vi "svx_Polar_Pane_Size.vi"(6 "Container bounds":T1, 7 "Display State In":T2={"Property Name"=[], "Container bounds"={"Width"=550, "Height"=250}, "Scale range"={"Maximum"=1.0, "Increment"=1.0}, "PointIdx"=0, "Marker list"=[], "Color settings"={"Arrow color"=16860, "Magnitude major grid"=13816530, "Magnitude minor grid"=16777216, "Phase grid"=13816530, "Phase scale marker text"=0}, "Magnitude scale name"="Magnitude", "Magnitude scale format string"="%#.2e", "MagnitudeScale:Visible"=TRUE, "MagnitudeScaleLabel:Visible"=TRUE, "PhaseScale:Visible"=TRUE, "Marker:Visible"=TRUE, "Cursor:Visible"=FALSE, "CursorName:Visible"=TRUE, "Autoscale"=TRUE, "Marker color"=16860, "Line color"=16711680, "Cursor color"=16711680, "Magnitude scale marker color"=0, "Plot.Line Style"=0, "Plot.Line Width"=0, "Plot.Point Style"=0, "Cursor.Line Style"=0, "Cursor.Line Width"=0, "Cursor.Point Style"=0, "Cursor.Style"=4, "Marker.Point Style"=2, "Point/fill color"=16711680, "Background color"=16777225, "Cursor name"="", "Cursor Release"=refnum, "Scale Range Change"=refnum, "data size(s)"=[], "Selectors:Visible"=TRUE, "Selector:ring Strings"={"Selector:Custom Strings"=FALSE, "Selector:Row Strings []"=[], "Selector:Column Strings []"=[], "User:Row Strings []"=[], "User:Column Strings []"=[]}, "Lock Cursor Info Position"=FALSE, "CursLoc"={"magnitude"=0.0, "phase"=0.0, "time/rev/RPM"=0.0}, "Plot Area:Position"={"Left"=0, "Top"=0}, "Plot Area:Size"={"Width"=0, "Height"=0}, "Marker.Style"=0, "Indication Arcs"=[], "Arc.Selector"=0, "customized marker"=[], "tree Width"=0, " Parents Tags"=[], "Children Tags"=[], "open?"=[], "index"=[{"row index"=0, "column index"=0}], "Label"="", "custom strings changed"=FALSE, "Owning VI"=refnum, "Legend BG color"=16777225, "Legend font color"=0, "column Width"=203, "attribute"=variant}, 8 "z scale graph Refnum":refnum<vi>, 9 "Plot Legend Refnum":refnum<vi>, 10 "Polar Plot Refnum in":refnum<vi>) -> (0 "z scale graph Refnum out":refnum<vi>, 1 "Plot Legend Refnum out":refnum<vi>, 2 "Polar Plot Refnum out":refnum<vi>, 5 "Display State out":T2={"Property Name"=[], "Container bounds"={"Width"=550, "Height"=250}, "Scale range"={"Maximum"=1.0, "Increment"=1.0}, "PointIdx"=0, "Marker list"=[], "Color settings"={"Arrow color"=16860, "Magnitude major grid"=13816530, "Magnitude minor grid"=16777216, "Phase grid"=13816530, "Phase scale marker text"=0}, "Magnitude scale name"="Magnitude", "Magnitude scale format string"="%#.2e", "MagnitudeScale:Visible"=TRUE, "MagnitudeScaleLabel:Visible"=TRUE, "PhaseScale:Visible"=TRUE, "Marker:Visible"=TRUE, "Cursor:Visible"=FALSE, "CursorName:Visible"=TRUE, "Autoscale"=TRUE, "Marker color"=16860, "Line color"=16711680, "Cursor color"=16711680, "Magnitude scale marker color"=0, "Plot.Line Style"=0, "Plot.Line Width"=0, "Plot.Point Style"=0, "Cursor.Line Style"=0, "Cursor.Line Width"=0, "Cursor.Point Style"=0, "Cursor.Style"=4, "Marker.Point Style"=2, "Point/fill color"=16711680, "Background color"=16777225, "Cursor name"="", "Cursor Release"=refnum, "Scale Range Change"=refnum, "data size(s)"=[], "Selectors:Visible"=TRUE, "Selector:ring Strings"={"Selector:Custom Strings"=FALSE, "Selector:Row Strings []"=[], "Selector:Column Strings []"=[], "User:Row Strings []"=[], "User:Column Strings []"=[]}, "Lock Cursor Info Position"=FALSE, "CursLoc"={"magnitude"=0.0, "phase"=0.0, "time/rev/RPM"=0.0}, "Plot Area:Position"={"Left"=0, "Top"=0}, "Plot Area:Size"={"Width"=0, "Height"=0}, "Marker.Style"=0, "Indication Arcs"=[], "Arc.Selector"=0, "customized marker"=[], "tree Width"=0, " Parents Tags"=[], "Children Tags"=[], "open?"=[], "index"=[{"row index"=0, "column index"=0}], "Label"="", "custom strings changed"=FALSE, "Owning VI"=refnum, "Legend BG color"=16777225, "Legend font color"=0, "column Width"=203, "attribute"=variant} caption="State")   [LabVIEW 2017, in "SVX Polar Plot.xctl"]
uses:
  <vilib>/addons/_XControls/Polar Plot/SVX Polar Plot.xctl
  <vilib>/addons/_XControls/Polar Plot/subVIs/svx_Polar_Plot_Internal_State.ctl
  <vilib>/addons/_XControls/Polar Plot/subVIs/svx_Polar_Indication_Arcs.ctl
  <vilib>/addons/_XControls/Polar Plot/subVIs/svx_Polar_Customized_Markers.ctl
  <vilib>/Utility/miscctls.llb/LVBoundsTypeDef.ctl
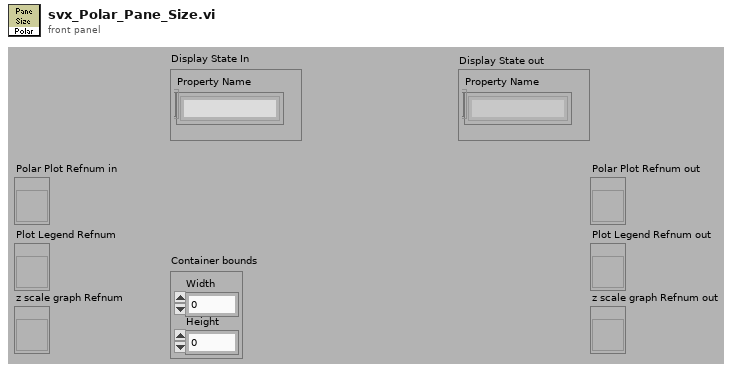
[diagram p1: front panel]
types:
  T1 = typedef "LVBoundsTypeDef.ctl" = cluster{"Width":u32, "Height":u32}
  T2 = typedef "SVX Polar Plot.xctl/svx_Polar_Plot_Internal_State.ctl" = cluster{"Property Name":string[], "Container bounds":cluster{"Width":u32, "Height":u32}, "Scale range":cluster{"Maximum":dbl, "Increment":dbl}, "PointIdx":i32, "Marker list":cluster{"Name":string, "Color":u32, "Style":u8, "Point Style":u8, "Name Visible":bool, "Allow Drag":bool, "Annotation Mode":u32, "Plot":i32, "Index":i32, "Position":cluster{"X":dbl, "Y":dbl}, "X Scale":u32, "Y Scale":u32, "Show Arrow":bool, "Lock Name":bool, "Plot Area":i32, "Label Offset":cluster{"X":dbl, "Y":dbl}}[], "Color settings":cluster{"Arrow color":u32, "Magnitude major grid":u32, "Magnitude minor grid":u32, "Phase grid":u32, "Phase scale marker text":u32}, "Magnitude scale name":string, "Magnitude scale format string":string, "MagnitudeScale:Visible":bool, "MagnitudeScaleLabel:Visible":bool, "PhaseScale:Visible":bool, "Marker:Visible":bool, "Cursor:Visible":bool, "CursorName:Visible":bool, "Autoscale":bool, "Marker color":u32, "Line color":u32, "Cursor color":u32, "Magnitude scale marker color":u32, "Plot.Line Style":i32, "Plot.Line Width":i32, "Plot.Point Style":i32, "Cursor.Line Style":i32, "Cursor.Line Width":i32, "Cursor.Point Style":i32, "Cursor.Style":i32, "Marker.Point Style":i32, "Point/fill color":u32, "Background color":u32, "Cursor name":string, "Cursor Release":refnum<user-event>, "Scale Range Change":refnum<user-event>, "data size(s)":i32[], "Selectors:Visible":bool, "Selector:ring Strings":cluster{"Selector:Custom Strings":bool, "Selector:Row Strings []":string[], "Selector:Column Strings []":string[], "User:Row Strings []":string[], "User:Column Strings []":string[]}, "Lock Cursor Info Position":bool, "CursLoc":cluster{"magnitude":dbl, "phase":dbl, "time/rev/RPM":dbl}, "Plot Area:Position":cluster{"Left":i32, "Top":i32}, "Plot Area:Size":cluster{"Width":u32, "Height":u32}, "Marker.Style":i32, "Indication Arcs":T3, "Arc.Selector":u16, "customized marker":T4, "tree Width":u32, " Parents Tags":string[], "Children Tags":string[], "open?":bool[], "index":cluster{"row index":i32, "column index":i32}[], "Label":string, "custom strings changed":bool, "Owning VI":refnum<vi>, "Legend BG color":u32, "Legend font color":u32, "column Width":u32, "attribute":variant}
  T3 = typedef "SVX Polar Plot.xctl/svx_Polar_Indication_Arcs.ctl" = cluster{"Name":string, "Start radius":dbl, "End radius":dbl, "Line Style":i32, "Line Width":i32, "Border color":u32, "Fill color":u32, "Start angle":i16, "End angle":i16, "Visible":bool}[]
  T4 = typedef "SVX Polar Plot.xctl/svx_Polar_Customized_Markers.ctl" = cluster{"Name":string, "Color":u32, "Style":u8, "Point Style":u8, "Name Visible":bool, "Allow Drag":bool, "Annotation Mode":u32, "Plot":i32, "Index":i32, "Position":cluster{"Magnitude":dbl, "Phase":dbl}, "X Scale":u32, "Y Scale":u32, "Show Arrow":bool, "Lock Name":bool, "Plot Area":i32, "Label Offset":cluster{"Magnitude":dbl, "Phase":dbl}}[]
  T5 = typedef "LVRectTypeDef.ctl" = cluster{"Left":i16, "Top":i16, "Right":i16, "Bottom":i16}
  T6 = cluster{"Left":i32, "Top":i32, "Right":i32, "Bottom":i32}
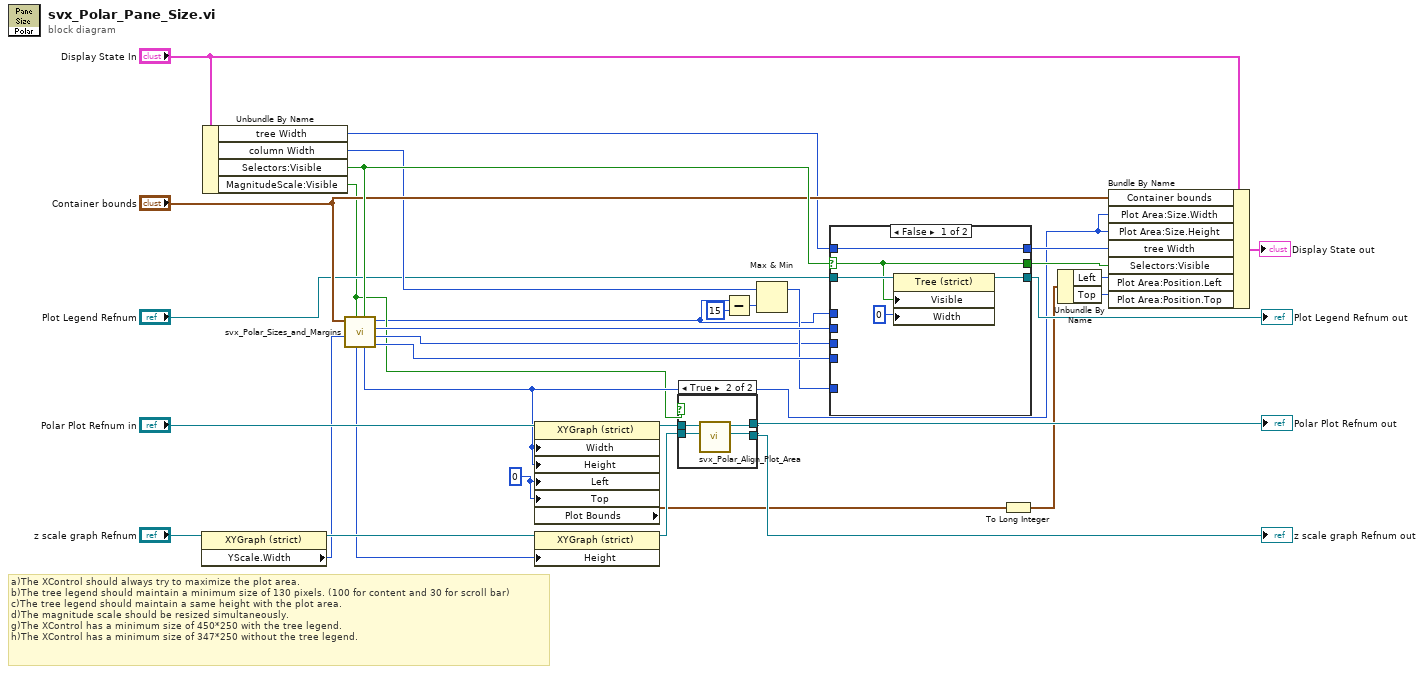
[diagram p0: block diagram]
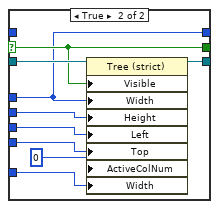
[diagram p2: hidden frame]
diagram:
  w32 = 0 ("Position:Left")
  # "a)The XControl should always try to maximize the plot area.\nb)The tree legend should maintain a minimum size of 130 pixels. (100 for content and 30 for scroll bar)\nc)The tree legend should maintain a same height with the plot area.\nd)The magnitude scale should be resized simultaneously.\ng)The XControl has a minimum size of 450*250 with the tree legend.\nh)The XControl has a minimum size of 347*250 without the tree legend."
  n1 = property class="XYGraph (strict)"(reference="z scale graph Refnum") -> (reference out=w31:refnum<vi>, "YScale.Width"=w9:u32)  [unwired: 1 in, 1 out]
  n2 = Unbundle By Name("Display State In") -> ("tree Width"=w7:u32, "column Width"=w6:u32, "Selectors:Visible"=w23:bool, "MagnitudeScale:Visible"=w3:bool)
  n3 = call <vilib>:"svx_Polar_Sizes_and_Margins.vi"("Selectors:Visible"=w23, "MagnitudeScale:Visible"=w3, "z scale width"=w9, "Container bounds"="Container bounds") -> ("tree top"=w16:u32, "tree left"=w10:u32, "tree height"=w18:u32, "tree width"=w2:u32, "plot area size"=w4:u32, "z-scale plot height"=w1:u32)  [unwired: 2 in]
  n4 = property on="Property Node" class="XYGraph (strict)"(reference="Polar Plot Refnum in", "Width"=w4, "Height"=w4, "Left"=w32, "Top"=w32) -> (reference out=w30:refnum<vi>, "Plot Bounds"=w26:T5)  [unwired: 1 in, 1 out]
  n5 = property class="XYGraph (strict)"(reference=w31, "Height"=w1) -> (reference out=w29:refnum<vi>)  [unwired: 1 in, 1 out]
  n6 = case shown="True" w3 {
    tunnel: w30 -> [w35 w39]
    tunnel: w29 -> [w34 w38]
    tunnel: [w34 w37] -> w28
    tunnel: [w35 w36] -> w19
    frame False {
    }
    frame True {
      n7 = call <vilib>:"svx_Polar_Align_Plot_Area.vi"("z scale graph ref in"=w38, "Polar Plot ref in"=w39) -> ("z scale graph ref out"=w37:refnum<vi>, "Polar Plot ref out"=w36:refnum<vi>)  [unwired: 8 in]
    }
  }
  "z scale graph Refnum out" <- w28
  "Polar Plot Refnum out" <- w19
  n8 = Subtract(x=w2, y=u32 15) -> (x-y=w21:u32)
  n9 = Max & Min(x=w6, y=w21) -> (max(x,y)=w11:u32)  [unwired: 1 out]
  n10 = case shown="False" w23 {
    selector: w23 -> [w41 w46]
    tunnel: w18 -> [_ w53]
    tunnel: [w43 w52] -> w24
    tunnel: w10 -> [_ w51]
    tunnel: "Plot Legend Refnum" -> [w44 w50]
    tunnel: w2 -> [_ w45]
    tunnel: w11 -> [_ w48]
    tunnel: [w41 w46] -> w17
    tunnel: w16 -> [_ w47]
    tunnel: w7 -> [w40 _]
    tunnel: [w40 w45] -> w8
    frame False {
      n11 = property class="Tree (strict)"(reference=w44, "Visible"=w41, "Width"=u32 0 ("Size:Width")) -> (reference out=w43:refnum<vi>)  [unwired: 1 in, 1 out]
    }
    frame True {
      n12 = property class="Tree (strict)"(reference=w50, "Visible"=w46, "Width"=w45, "Height"=w53, "Left"=w51, "Top"=w47, "ActiveColNum"=0 ("Active Cell:Active Column Number"), "Width"=w48) -> (reference out=w52:refnum<vi>)  [unwired: 1 in, 1 out]
    }
  }
  "Plot Legend Refnum out" <- w24
  n13 = To Long Integer(number=w26) -> (32bit integer=w12:T6)
  n14 = Unbundle By Name(w12) -> ("Left"=w14:i32, "Top"=w13:i32)
  n15 = Bundle By Name(cluster="Display State In", "Container bounds"="Container bounds", "Plot Area:Size.Width"=w4, "Plot Area:Size.Height"=w4, "tree Width"=w8, "Selectors:Visible"=w17, "Plot Area:Position.Left"=w14, "Plot Area:Position.Top"=w13) -> (→"Display State out":T2)
